vi "Graph Plot as Spline.vi"() -> ()   [LabVIEW 2018]
uses:
  <vilib>/Analysis/1siggen.llb/Ramp Pattern by Samples.vi
  <vilib>/Analysis/NI_AALBase.lvlib
  <vilib>/gmath/NI_Gmath.lvlib
panel:
  in  "Stop":bool
  in  "Interpolation Method":i32(ring)=3 items=["nearest", "linear", "spline", "cubic Hermite", "Lagrange"]
  out "XY Graph":cluster{"xi used":dbl[], "yi":dbl[]}[](graph)=[{"xi used"=[-50.0, -49.173228346456696, -48.346456692913385, -47.51968503937008, -46.69291338582677, -45.86614173228347, -45.039370078740156, -44.21259842519685, -43.38582677165354, -42.55905511811024, -41.73228346456693, -40.90551181102362, -40.07874015748031, -39.25196850393701, -38.425196850393704, -37.59842519685039, -36.77165354330709, -35.94488188976378, -35.118110236220474, -34.29133858267717, -33.46456692913386, -32.63779527559055, -31.811023622047244, -30.984251968503937, -30.15748031496063, -29.330708661417322, -28.503937007874015, -27.67716535433071, -26.850393700787404, -26.023622047244096, -25.19685039370079, -24.37007874015748, -23.543307086614174, -22.716535433070867, -21.88976377952756, -21.062992125984252, -20.236220472440944, -19.409448818897637, -18.582677165354333, -17.755905511811022, -16.92913385826772, -16.102362204724407, -15.275590551181104, -14.4488188976378, -13.622047244094489, -12.795275590551185, -11.968503937007874, -11.14173228346457, -10.31496062992126, -9.488188976377955, -8.661417322834644, -7.834645669291341, -7.00787401574803, -6.181102362204726, -5.354330708661422, -4.527559055118111, -3.7007874015748072, -2.8740157480314963, -2.0472440944881924, -1.2204724409448815, -0.39370078740157766, 0.4330708661417333, 1.2598425196850371, 2.086614173228348, 2.913385826771652, 3.7401574803149558, 4.566929133858267, 5.3937007874015706, 6.2204724409448815, 7.047244094488185, 7.874015748031496, 8.7007874015748, 9.527559055118111, 10.354330708661415, 11.181102362204726, 12.00787401574803, 12.834645669291334, 13.661417322834644, 14.488188976377955, 15.31496062992126, 16.141732283464563, 16.968503937007867, 17.795275590551185, 18.62204724409449, 19.448818897637793, 20.275590551181097, 21.1023622047244, 21.92913385826772, 22.755905511811022, 23.582677165354326, 24.40944881889763, 25.236220472440948, 26.062992125984252, 26.889763779527556, 27.71653543307086, 28.543307086614178, 29.37007874015748, 30.196850393700785, 31.02362204724409, 31.850393700787393, 32.67716535433071, 33.503937007874015, 34.33070866141732, 35.15748031496062, 35.98425196850394, 36.811023622047244, 37.63779527559055, 38.46456692913385, 39.291338582677156, 40.118110236220474, 40.94488188976378, 41.77165354330708, 42.598425196850386, 43.425196850393704, 44.25196850393701, 45.07874015748031, 45.905511811023615, 46.73228346456693, 47.55905511811024, 48.38582677165354, 49.212598425196845, 50.03937007874015, 50.86614173228347, 51.69291338582677, 52.519685039370074, 53.34645669291338, 54.173228346456696, 55.0], "yi"=[4.0, 3.6539734024349952, 3.3242914044883207, 3.010558572298248, 2.712379472003038, 2.429358669740962, 2.161100731650282, 1.9072102238692672, 1.6672917125361804, 1.440949763789292, 1.2277889437668654, 1.0274138186071649, 0.8394289544484597, 0.6634389174290161, 0.49904827368709936, 0.34586158936097444, 0.20348343058890883, 0.07151836350916829, -0.05042904573998097, -0.16275423102027187, -0.26585262619344174, -0.3601196651212213, -0.4459507816653421, -0.5237414096875437, -0.5938869830495568, -0.6567829356131147, -0.7128247012399527, -0.7624077137918048, -0.8059274071304037, -0.8437792151174852, -0.8763585716147801, -0.9040609104840254, -0.9272816655869534, -0.9464162707852966, -0.9618601599407919, -0.9740087669151718, -0.9832575255701697, -0.9900018697675197, -0.9946372333689544, -0.9975590502362097, -0.9991627542310182, -0.9998437792151167, -0.9999975590502368, -0.9697342727942082, -0.816054006820576, -0.5424481502140266, -0.16018067498519506, 0.3194844468552722, 0.8852832432967437, 1.5259517423285698, 2.2302259719401216, 2.9868419601207474, 3.78453573485982, 4.612043324146687, 5.4581007559707135, 6.31144405832127, 7.160809259187701, 7.994932386559379, 8.802549468425651, 9.572396532775894, 10.29320960759945, 10.953724720885695, 11.542677900623978, 12.049457685893588, 12.534253861173948, 13.037062785478291, 13.550788007776545, 14.068333077038627, 14.582601542234471, 15.086496952333995, 15.572922856307132, 16.0347828031238, 16.464980341753932, 16.856419021167444, 17.202002390334272, 17.49463399822433, 17.727217393807553, 17.892656126053865, 17.983853743933185, 17.988957143268618, 17.858931487055887, 17.592666508167664, 17.20287787672032, 16.70228126283024, 16.103592336613808, 15.4195267681874, 14.662800227667393, 13.846128385170154, 12.982226910812091, 12.083811474709568, 11.163597746978965, 10.234301397736651, 9.30863809709903, 8.399323515182468, 7.5190733221033454, 6.680603187978026, 5.896628782922921, 5.179865777054392, 4.5430298404888205, 3.9988366433425853, 3.560001855732061, 3.2392411477736403, 3.049270189583689, 3.0029911953490256, 3.107503199327237, 3.3323400783758936, 3.637958446321611, 3.984814916991003, 4.333366104210683, 4.6440686218072695, 4.877379083607367, 4.993754103437594, 4.987921257074259, 4.931250125715301, 4.827749009828728, 4.6769328414776385, 4.478316552725129, 4.231415075634295, 3.9357433422682435, 3.590816284690068, 3.1961488349628673, 2.75125592514974, 2.255652487313775, 1.7088534535180893, 1.110373755825771, 0.45972832629992055, -0.24356790299637776, -1.0]}, {"xi used"=[-50.0, -15.0, 2.0, 15.0, 35.0, 42.0, 55.0], "yi"=[4.0, -1.0, 12.0, 18.0, 3.0, 5.0, -1.0]}]
  in  "Y":dbl[](array[numeric])=[4.0, -1.0, 12.0, 18.0, 3.0, 5.0, -1.0]
  in  "X":dbl[](array[numeric])=[-50.0, -15.0, 2.0, 15.0, 35.0, 42.0, 55.0]
  # "This vi demonstrations how to smooth the representation of a curve in a graph plot"
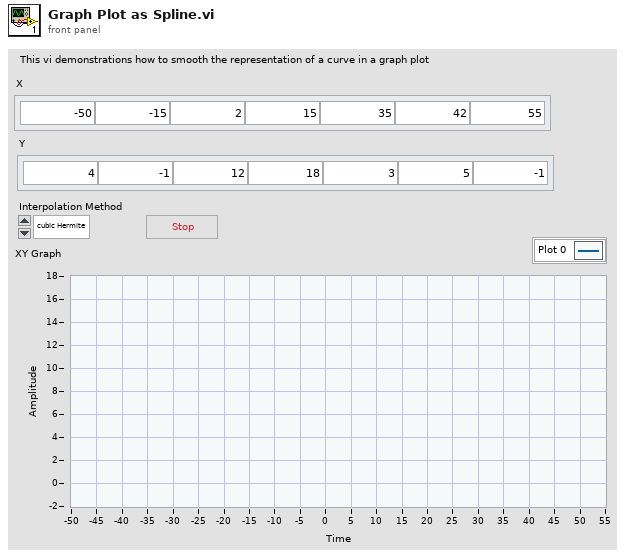
[diagram p1: front panel]
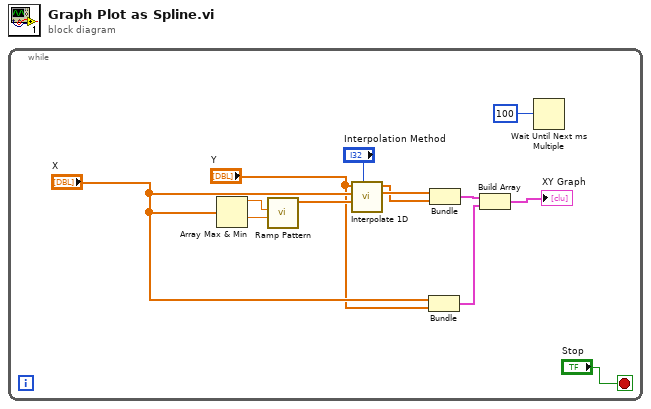
[diagram p0: block diagram]
diagram:
  n1 = while {
    stop <- "Stop" stop-if-true
    n2 = Array Max & Min(array="X") -> (max value=w13:dbl, min value=w12:dbl)  [unwired: 2 out]
    n3 = call-poly <vilib>:"Ramp Pattern.vi"("start"=w12, "end"=w13) -> ("Ramp Pattern"=w11:dbl[])  [unwired: 8 in, 1 out]
    n4 = call <vilib>:"Interpolate 1D.vi"("method"="Interpolation Method", "xi"=w11, "X"="X", "Y"="Y") -> ("xi used"=w10:dbl[], "yi"=w9:dbl[])  [unwired: 5 in, 1 out]
    n5 = Bundle("X"="X", "Y"="Y") -> (w3:cluster{"X":dbl[], "Y":dbl[]})  [unwired: 1 in]
    n6 = Bundle("xi used"=w10, "yi"=w9) -> (w8:cluster{"xi used":dbl[], "yi":dbl[]})  [unwired: 1 in]
    n7 = Build Array(w8, w3) -> (→"XY Graph":cluster{"X":dbl[], "Y":dbl[]}[])
    n8 = Wait Until Next ms Multiple(millisecond multiple=100) -> ()  [unwired: 1 out]
  }
